vi "Query Gate Width.vi"(8 "error in (no error)":errorcluster, 10 "Gate (def: A)":T1, 11 "VISA resource name":refnum<visa-resource-name>) -> (0 "error out":errorcluster, 2 "width (s)":dbl, 3 "VISA resource name out":refnum<visa-resource-name>)   [LabVIEW 2017, in "SR400.lvlib"]
doc: "The GW command sets and reads the gate widths.\ni = 0 or 1 designates A gate or B gate and is\nrequired. If t is included, the selected gate width is\nset to t seconds where 0.005E-6 <= t <= 999.2E-3.\nThe resolution is variable depending upon the 4\nmost significant digits of t.\n4 most significant digits resolution in 4th digit\n1000 to 2048 1 (1001,1002,1003,...)\n2048 to 4096 2\n4096 to 8192 4\n8192 to 9992 8 (8192,8200,8208,...)\nFor example, near 10.00 ìs, the allowed values of\nt are 9.984 ìs, 9.992 ìs, 10.00 ìs, 10.01 ìs, etc.\nBelow 1.000 ìs, the resolution is 1 ns. Almost any\nvalue of t may be sent and the SR400 will round to\nthe nearest allowed value. If t is absent, the\nselected gate width is returned. The gate width\nmay be read and set regardless of the gate mode. If\nthe mode is CW, the gate remains continuous. If\nthe mode is FIXED or SCAN, the gate width is\nadjusted immediately.\nNOTE\nChanging the gate delay or width may cause some\ngates to be missed or shortened. Changing gate\nparameters while counting may therefore cause\nbad data to be collected. It is recommended that\nthe counters be paused before changing gate\nvalues and then started again."
uses:
  SR400.lvlib
  Typedefs.llb/Gate.ctl
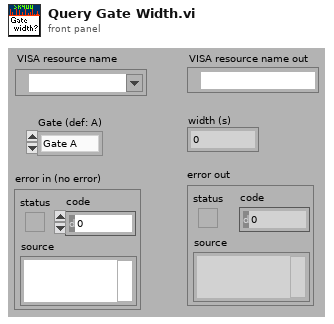
[diagram p1: front panel]
types:
  T1 = typedef "SR400.lvlib/Gate.ctl" = enum16{"Gate A", "Gate B"}
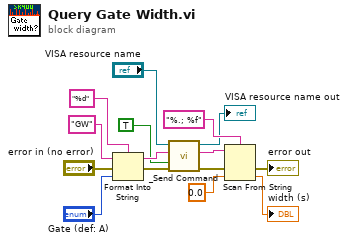
[diagram p0: block diagram]
diagram:
  n1 = Format Into String(format string="%d", initial string="GW" ("command"), error in="error in (no error)", "Gate (def: A)") -> (resulting string=w6:string, error out=w5:errorcluster)
  n2 = call "_Send Command.vi"("error in (no error)"=w5, "Query? (F)"=TRUE, "Command"=w6, "VISA resource name"="VISA resource name") -> ("error out"=w2:errorcluster, "Response"=w3:string, "VISA resource name out"=→"VISA resource name out":refnum<visa-resource-name>)  [unwired: 5 out]
  n3 = Scan From String(format string="%.; %f", input string=w3, error in=w2, default 1=0.0 ("default value 1")) -> (error out=→"error out":errorcluster, output 1=→"width (s)":dbl)  [unwired: 1 in, 2 out]
